vi "Configure Modulation Low Level (PWM Deviation).vi"(8 "error in":errorcluster, 10 "Pulse Width Deviation (10 us)":dbl=1e-05, 11 "VISA resource name":refnum<visa-resource-name>) -> (0 "error out":errorcluster, 3 "VISA resource name out":refnum<visa-resource-name>)   [LabVIEW 2017, in "Keithley 3390.lvlib"]
doc: "Sets the pulse width deviation for the pulse width modulation technique. The width deviation represents the peak variation in the pulse width of the modulation output based on that of the original pulse carrier waveform."
uses:
  Keithley 3390.lvlib
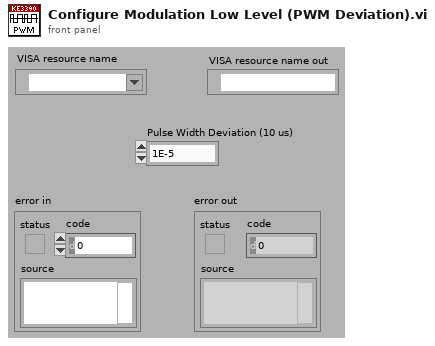
[diagram p1: front panel]
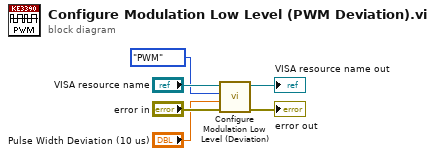
[diagram p0: block diagram]
diagram:
  n1 = call "Configure Modulation Low Level (Deviation).vi"("error in (no error)"="error in", "Deviation"="Pulse Width Deviation (10 us)", "Modulation (FM)"=enum16{"FM", "PM", "PWM"}."PWM" ("Modulation (0: FM)"), "VISA resource name"="VISA resource name") -> ("error out"=→"error out":errorcluster, "VISA resource name out"=→"VISA resource name out":refnum<visa-resource-name>)  [unwired: 6 in]
